vi "DriverStationGetInstructions.vi"   [LabVIEW 2019]
uses:
  refnums.vi
  <vilib>/Rock Robotics/WPI/Utilities/WPI_GetSetVariantRefNum.vi
  dsinstructions.vi
types:
  T1 = typedef "WPI_JoystickDevRef.ctl" = cluster{"Device":T2}
  T2 = typedef "WPI_JoystickDeviceEnum.ctl" = enum16{"USB 0", "USB 1", "USB 2", "USB 3", "USB 4", "USB 5"}
  T3 = enum16{"Center", "North", "NorthWest", "West", "SouthWest", "South", "SouthEast", "East", "NorthEast"}
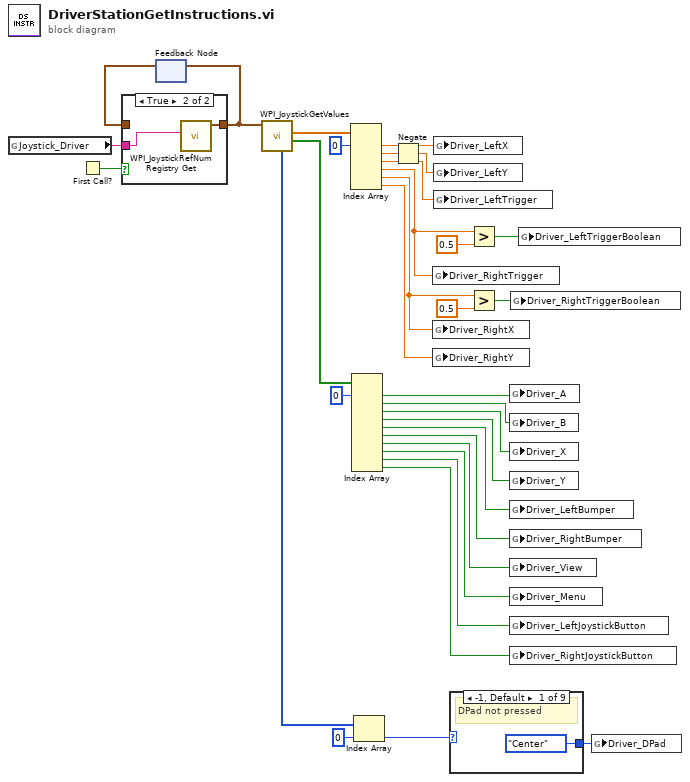
[diagram p0: block diagram]
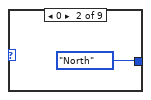
[diagram p2: hidden frame]
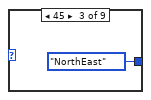
[diagram p3: hidden frame]
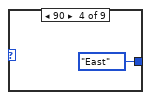
[diagram p4: hidden frame]
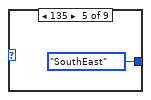
[diagram p5: hidden frame]
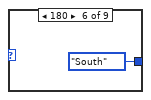
[diagram p6: hidden frame]
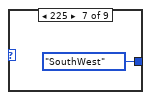
[diagram p7: hidden frame]
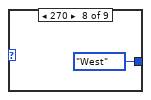
[diagram p8: hidden frame]
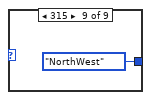
[diagram p9: hidden frame]
diagram:
  n1 = global read "refnums.vi" "Joystick_Driver"() -> (w30:string)
  n2 = First Call?() -> (First Call?: T/F=w33:bool)
  n3 = feedback #1() -> (w32:T1)  [unwired: 1 in]
  n4 = case shown="True" w33 {
    tunnel: [w34 w36] -> w31
    tunnel: w32 -> [w34 _]
    tunnel: w30 -> [_ w35]
    frame False {
    }
    frame True {
      n5 = call <vilib>:"WPI_JoystickRefNum Registry Get.vi"("refnum name"=w35) -> ("JoystickDevRef"=w36:T1)  [unwired: 9 in, 1 out]
    }
  }
  n6 = feedback-in #1(w31) -> ()
  n7 = call <vilib>:"WPI_JoystickGetValues.vi"("JoystickDevRef"=w31) -> ("Buttons"=w28:bool[], "Axes"=w29:dbl[], "POVs"=w25:i16[])  [unwired: 6 in, 2 out]
  n8 = Index Array(array=w29, index #1=0 ("index")) -> (element #1=w13:dbl, element #2=w12:dbl, element #3=w11:dbl, element #4=w6:dbl, element #5=w3:dbl, element #6=w10:dbl)  [unwired: 5 in]
  n9 = Index Array(array=w28, index #1=0 ("index")) -> (element #1=w23:bool, element #2=w22:bool, element #3=w21:bool, element #4=w20:bool, element #5=w19:bool, element #6=w18:bool, element #7=w17:bool, element #8=w16:bool, element #9=w15:bool, element #10=w14:bool)  [unwired: 9 in]
  n10 = Index Array(array=w25, index=0) -> (element=w2:i16)
  n11 = Negate(x=w12) -> (-x=w9:dbl)
  n12 = global write "dsinstructions.vi" "Driver_RightTrigger"(w6) -> ()
  n13 = global write "dsinstructions.vi" "Driver_RightX"(w3) -> ()
  n14 = global write "dsinstructions.vi" "Driver_RightY"(w10) -> ()
  n15 = global write "dsinstructions.vi" "Driver_LeftX"(w13) -> ()
  n16 = global write "dsinstructions.vi" "Driver_LeftY"(w9) -> ()
  n17 = global write "dsinstructions.vi" "Driver_LeftTrigger"(w11) -> ()
  n18 = case shown="-1, Default" w2 {
    tunnel: [T3."Center" T3."North" T3."NorthEast" T3."East" T3."SouthEast" T3."South" T3."SouthWest" T3."West" T3."NorthWest"] -> w1
    frame -1, Default {
      # "DPad not pressed"
    }
    frame 0 {
    }
    frame 45 {
    }
    frame 90 {
    }
    frame 135 {
    }
    frame 180 {
    }
    frame 225 {
    }
    frame 270 {
    }
    frame 315 {
    }
  }
  n19 = Greater?(x=w6, y=0.5) -> (0:w8:bool)
  n20 = Greater?(x=w3, y=0.5) -> (0:w5:bool)
  n21 = global write "dsinstructions.vi" "Driver_A"(w23) -> ()
  n22 = global write "dsinstructions.vi" "Driver_B"(w22) -> ()
  n23 = global write "dsinstructions.vi" "Driver_X"(w21) -> ()
  n24 = global write "dsinstructions.vi" "Driver_Y"(w20) -> ()
  n25 = global write "dsinstructions.vi" "Driver_LeftBumper"(w19) -> ()
  n26 = global write "dsinstructions.vi" "Driver_RightBumper"(w18) -> ()
  n27 = global write "dsinstructions.vi" "Driver_View"(w17) -> ()
  n28 = global write "dsinstructions.vi" "Driver_Menu"(w16) -> ()
  n29 = global write "dsinstructions.vi" "Driver_LeftJoystickButton"(w15) -> ()
  n30 = global write "dsinstructions.vi" "Driver_RightJoystickButton"(w14) -> ()
  n31 = global write "dsinstructions.vi" "Driver_RightTriggerBoolean"(w5) -> ()
  n32 = global write "dsinstructions.vi" "Driver_LeftTriggerBoolean"(w8) -> ()
  n33 = global write "dsinstructions.vi" "Driver_DPad"(w1) -> ()
